vi "2D Size - String.vi"(8 "size(s)":i32[](array[numeric])) -> (0 "size (string)":variant)   [LabVIEW 2014]
doc: "<B>Copyrights</B>: (c) 2015 MHWirth. All rights reserved.\n\nThis subVI gets the size of a 2D array and make an string for the size."
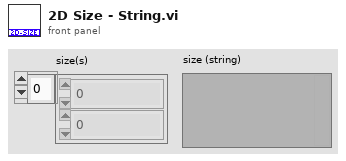
[diagram p1: front panel]
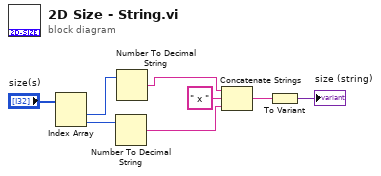
[diagram p0: block diagram]
diagram:
  n1 = Index Array(array="size(s)") -> (element #1=w7:i32, element #2=w6:i32)  [unwired: 2 in]
  n2 = Number To Decimal String(number=w6) -> (decimal integer string=w3:string)  [unwired: 1 in]
  n3 = Number To Decimal String(number=w7) -> (decimal integer string=w4:string)  [unwired: 1 in]
  n4 = Concatenate Strings(w4, " x " ("string"), w3) -> (w2:string)
  n5 = To Variant(anything=w2) -> (Variant=→"size (string)":variant)
